vi "Type Dict LV.vi"() -> ()   [LabVIEW 2020, in "LV Tiff.lvlib"]
uses:
  <vilib>/Utility/Data Type/Type Definitions/Data Type.ctl
  Tiff Data Type.ctl
  LV Tiff.lvlib
  <vilib>/Utility/Data Type/NI_Data Type.lvlib
panel:
  out "map":map{T1, T2}(c390)
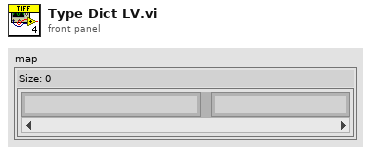
[diagram p1: front panel]
types:
  T1 = typedef "NI_Data Type.lvlib/Data Type.ctl" = enum8{"Invalid Type", "Void", "I8", "I16", "I32", "I64", "U8", "U16", "U32", "U64", "Single Float", "Double Float", "Extended Float", "Single Complex", "Double Complex", "Extended Complex", "Enum U8", "Enum U16", "Enum U32", "Enum U64", "Single Float With Unit", "Double Float With Unit", "Extended Float With Unit", "Single Complex with Unit", "Double Complex with Unit", "Extended Complex with Unit", "Boolean", "String", "Path", "Picture", "Tag", "Array", "Cluster", "Variant", "LV Variant", "Waveform", "Timestamp", "Digital Waveform", "Digital Data", "ExpressData", "Refnum", "External Data", "VI", "Poly VI", "LabVIEW Class Instance", "Fixed Point", "Set Collection", "Map Collection"}
  T2 = typedef "LV Tiff.lvlib/Tiff Data Type.ctl" = enum16{"Null", "BYTE", "ASCII", "SHORT", "LONG", "RATIONAL", "SBYTE", "UNDEFINE", "SSHORT", "SLONG", "SRATIONAL", "FLOAT", "DOUBLE"}
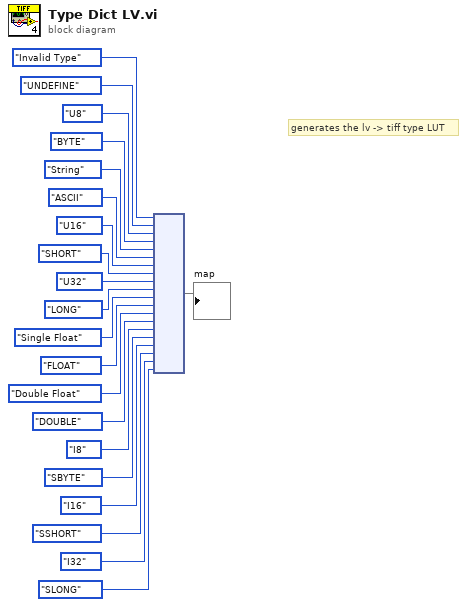
[diagram p0: block diagram]
diagram:
  # "generates the lv -> tiff type LUT"
  n1 = node(Data_Type."Invalid Type" ("type"), Tiff_Data_Type."UNDEFINE" ("DataType"), Data_Type."U8" ("key"), Tiff_Data_Type."BYTE" ("value"), Data_Type."String" ("key"), Tiff_Data_Type."ASCII" ("value"), Data_Type."U16" ("key"), Tiff_Data_Type."SHORT" ("value"), Data_Type."U32" ("key"), Tiff_Data_Type."LONG" ("value"), Data_Type."Single Float" ("key"), Tiff_Data_Type."FLOAT" ("value"), Data_Type."Double Float" ("key"), Tiff_Data_Type."DOUBLE" ("value"), Data_Type."I8" ("key"), Tiff_Data_Type."SBYTE" ("value"), Data_Type."I16" ("key"), Tiff_Data_Type."SSHORT" ("value"), Data_Type."I32" ("key"), Tiff_Data_Type."SLONG" ("value")) -> (→"map":map{T1, T2})
